vi "Set Input 3 Path.vi"(8 "error in (no error)":errorcluster, 10 "Input Path":string, 11 "Item Ref in":T1 format="%.0x") -> (0 "error out":errorcluster)   [LabVIEW 2019]
uses:
  <vilib>/NI VeriStand/Custom Device API/Custom Device API.lvlib
  Shared/Constants.vi
  Shared/Software Multi-Plex Shared.lvlib
  <vilib>/NI VeriStand/Custom Device API/Set Item Property (String).vi
  <vilib>/NI VeriStand/Custom Device API/Custom Device Item Ref.ctl
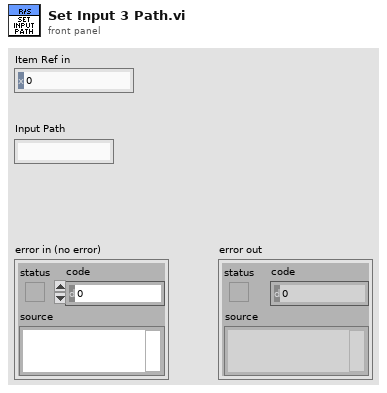
[diagram p1: front panel]
types:
  T1 = typedef "Custom Device API.lvlib/Custom Device Item Ref.ctl" = u64
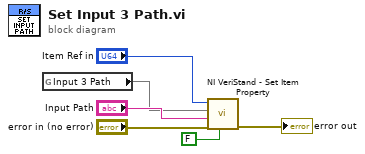
[diagram p0: block diagram]
diagram:
  n1 = global read "Constants.vi" "Input 3 Path"() -> (w1)
  n2 = call-poly <vilib>:"NI VeriStand - Set Item Property.vi"("Binary String (T)"=FALSE, "error in (no error)"="error in (no error)", "Value"="Input Path", "Property Name"=w1, "Item Ref in"="Item Ref in") -> ("error out"=→"error out":errorcluster)  [unwired: 4 in, 2 out]
